vi "Handle Step.vi"(0 "reference in":refnum<class "Stand.lvclass">, 11 "error in (no error)":errorcluster) -> (4 "reference out":refnum<class "Stand.lvclass">, 15 "error out":errorcluster)   [LabVIEW 2019, in "Stand.lvclass"]
uses:
  Stand.lvclass
  Stand.lvclass/Stand.ctl
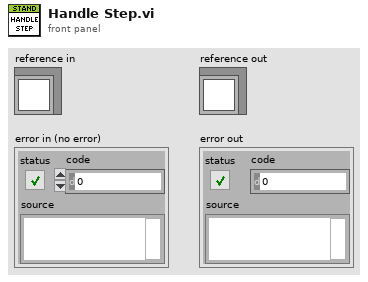
[diagram p1: front panel]
types:
  T1 = typedef "Step_Name.ctl" = enum16{"Filling DUT", "Filling Chamber", "Pressure Up DUT", "Abrupt Pressure Release DUT", "Smooth Pressure Release DUT", "Pressure Up Chamber", "Abrupt Pressure Release Chamber", "Smooth Pressure Release Chamber", "Measuring leakage sensor 41.3", "Measuring leakage burette 42", "IDLE", "Low Pressure DUT", "Low Pressure Chamber"}
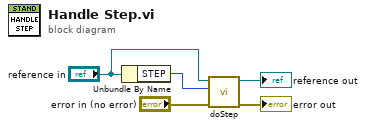
[diagram p0: block diagram]
diagram:
  n1 = Unbundle By Name("reference in") -> ("STEP"=w5:T1)
  n2 = call "doStep.vi"("error in (no error)"="error in (no error)", "stepName"=w5, "Stand in"="reference in") -> ("error out"=→"error out":errorcluster, "Stand out"=→"reference out":refnum<class "Stand.lvclass">)  [unwired: 7 in]
